vi "FFTIni2.vi"() -> (1 "xyz_o":dbl[][](array[numeric]))   [LabVIEW 2013]
uses:
  <vilib>/Utility/file.llb/Read From Spreadsheet File (DBL).vi
panel:
  out "initialized array":dbl[](array[numeric])
  in  "file path (use dialog)":path=path "C:/JK/posi2.txt"
  out "y_o":dbl[](array[numeric])
  out "all rows":dbl[][](array[numeric]) format="%0.3f"
  out "x_o":dbl[](array[numeric])
  out "array w/ subset deleted":dbl[][](array[numeric])
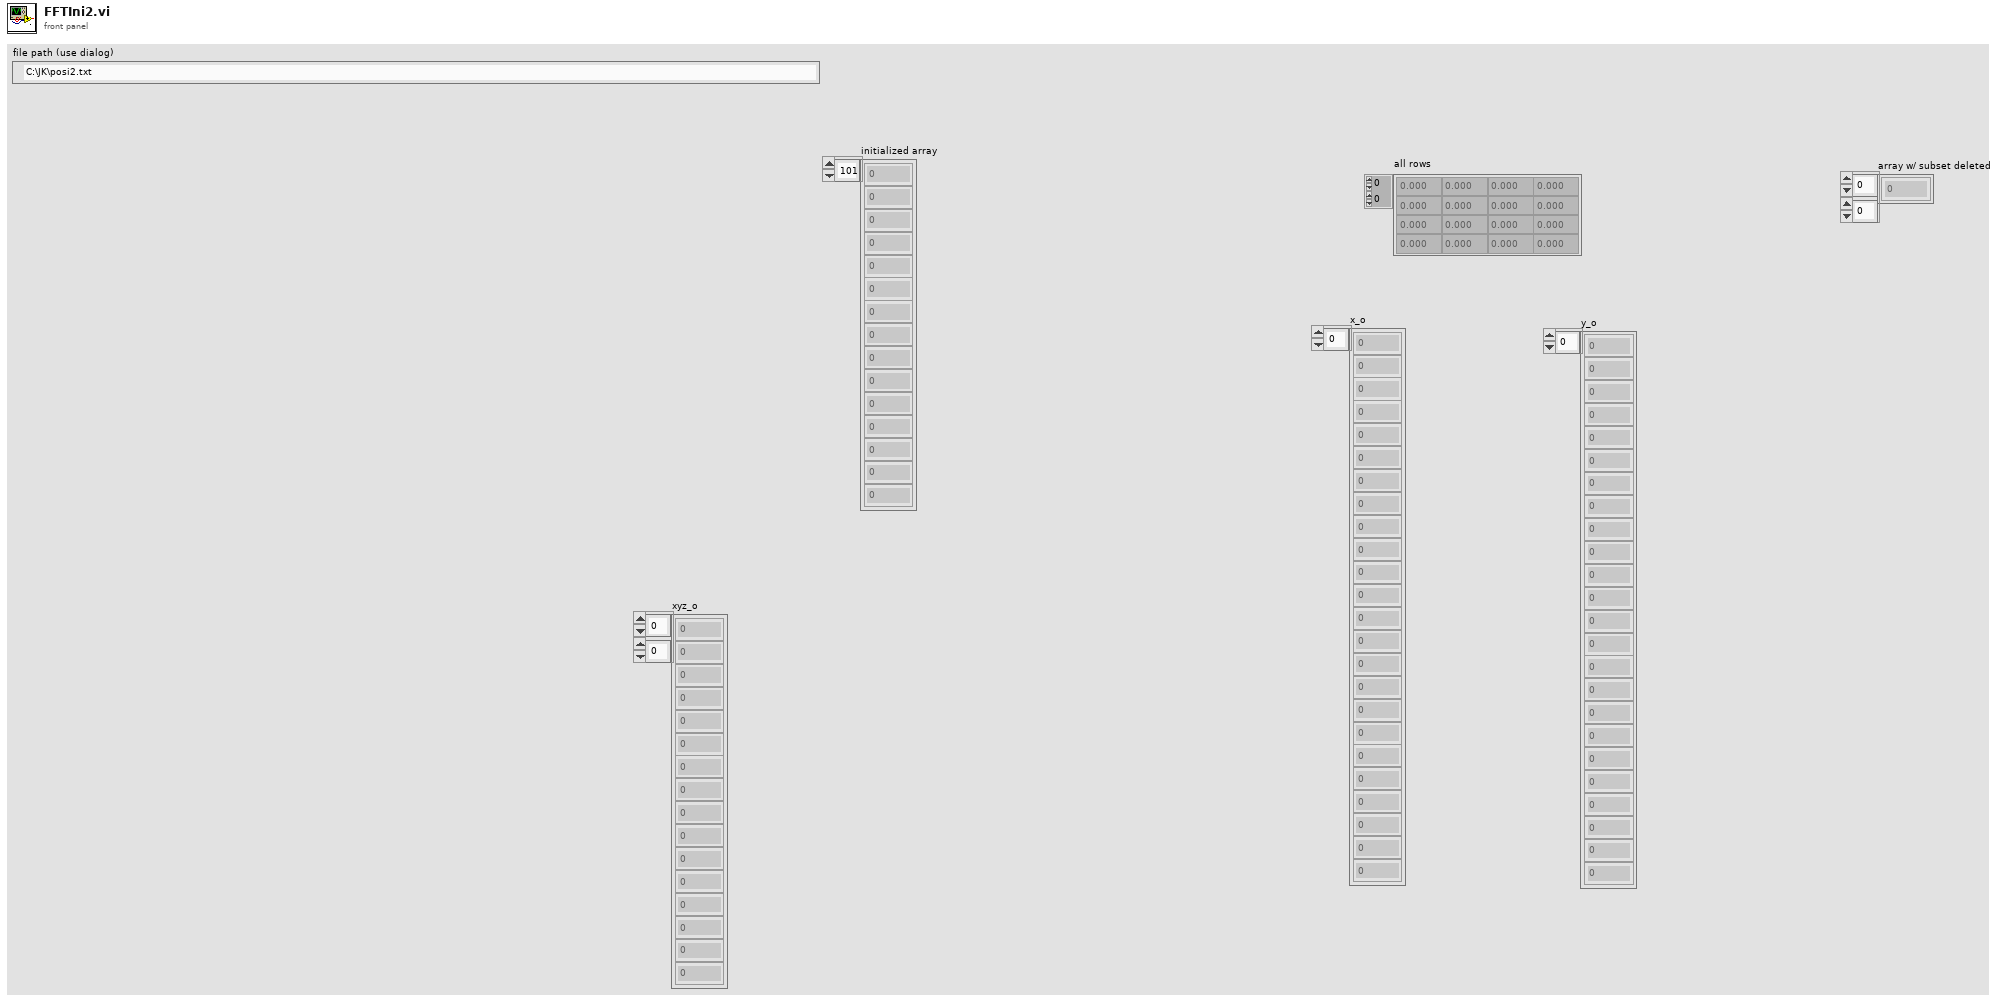
[diagram p1: front panel]
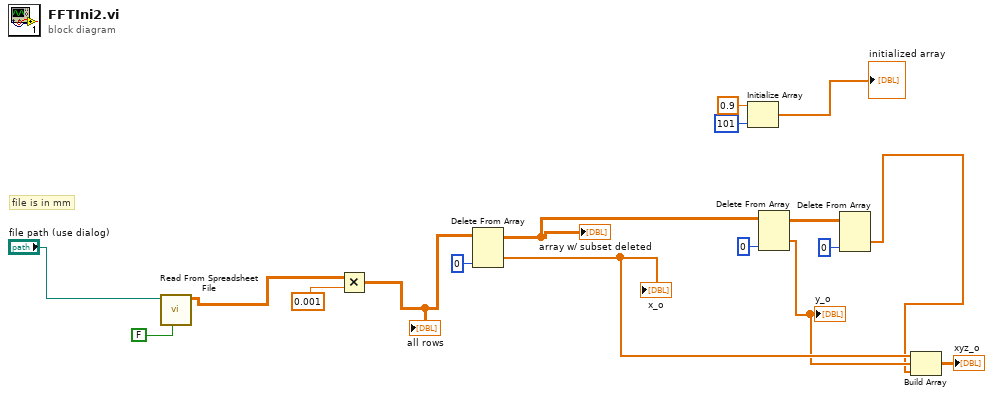
[diagram p0: block diagram]
diagram:
  # "file is in mm"
  n1 = call-poly <vilib>:"Read From Spreadsheet File.vi"("transpose (no:F)"=FALSE, "file path (dialog if empty)"="file path (use dialog)") -> ("all rows"=w8:dbl[][])  [unwired: 5 in, 4 out]
  n2 = Multiply(x=w8, y=0.001) -> (x*y=w12:dbl[][])
  "all rows" <- w12
  n3 = Delete From Array(array=w12, index (col)=0 ("disabled index (col)")) -> (deleted portion=w10:dbl[], array with subset deleted=w15:dbl[][])  [unwired: 2 in]
  "array w/ subset deleted" <- w15
  "x_o" <- w10
  n4 = Initialize Array(0.9 ("element"), 101 ("dimension size")) -> (→"initialized array":dbl[])
  n5 = Delete From Array(array=w15, index (col)=0) -> (deleted portion=w9:dbl[], array with subset deleted=w14:dbl[][])  [unwired: 2 in]
  "y_o" <- w9
  n6 = Delete From Array(array=w14, index (col)=0 ("disabled index (col)")) -> (deleted portion=w1:dbl[])  [unwired: 2 in, 1 out]
  n7 = Build Array(w10, w9, w1) -> (→"xyz_o":dbl[][])
